vi "ICR_Setup_Sequence.vi"(8 "error in (no error)":errorcluster, 9 "QMH UI Cluster":variant, 11 "QMH ICR Cluster":T1) -> (0 "error out":errorcluster, 3 "QMH ICR Cluster":T1)   [LabVIEW 2024]
doc: "This VI updates the indicators of the ICR panel according to the parameters setup by the user and the controls in the UI main panel.\n\n1. The indicators are passed by reference through the QMH ICR Cluster.\n2. Their values are updated with the QMH UI Cluster parameters.\n3. The QMH ICR Cluster given in output contains the updated indicators."
uses:
  controls/QMH_ICR_Cluster.ctl
  controls/HARDWARE_Resources.ctl
  controls/PROCESSING_Inputs.ctl
  controls/LOOPS_Inputs.ctl
  controls/OPO_Inputs.ctl
  controls/QMH_UI_Cluster.ctl
  controls/QMH_UI_References.ctl
  controls/QMH_UI_Report.ctl
  controls/QMH_UI_Command.ctl
  controls/QMH_ICR_Command.ctl
  controls/QMH_Status.ctl
  controls/EXPERT_Inputs.ctl
  controls/DIGIT_5122_Inputs.ctl
  <instrlib>/niScope/Controls/niScope trigger source.ctl
  controls/HSDIO_6541_Inputs.ctl
  <instrlib>/niHSDIO/niHSDIO.llb/niHSDIO_ctl Trigger Source Values (Ring).ctl
  controls/SOFTWARE_Inputs.ctl
  controls/AO_6711_Inputs.ctl
  controls/AWG_5421_Inputs.ctl
  <instrlib>/niFgen/niFgen.llb/niFgen_ctl Trigger Source Values (Ring).ctl
  controls/XML_Inputs.ctl
  controls/SEQUENCE_Inputs.ctl
  controls/EXCIT_Inputs.ctl
  controls/DATA_Inputs.ctl
  controls/TIMING_Inputs.ctl
  controls/TRAPPING_Inputs.ctl
  controls/EXPERT_Path_Selector.ctl
  controls/EXPERIMENT_Inputs.ctl
  controls/LASER_Inputs.ctl
  controls/LAMP_Inputs.ctl
  controls/GAS_Inputs.ctl
  Global_Variables.vi
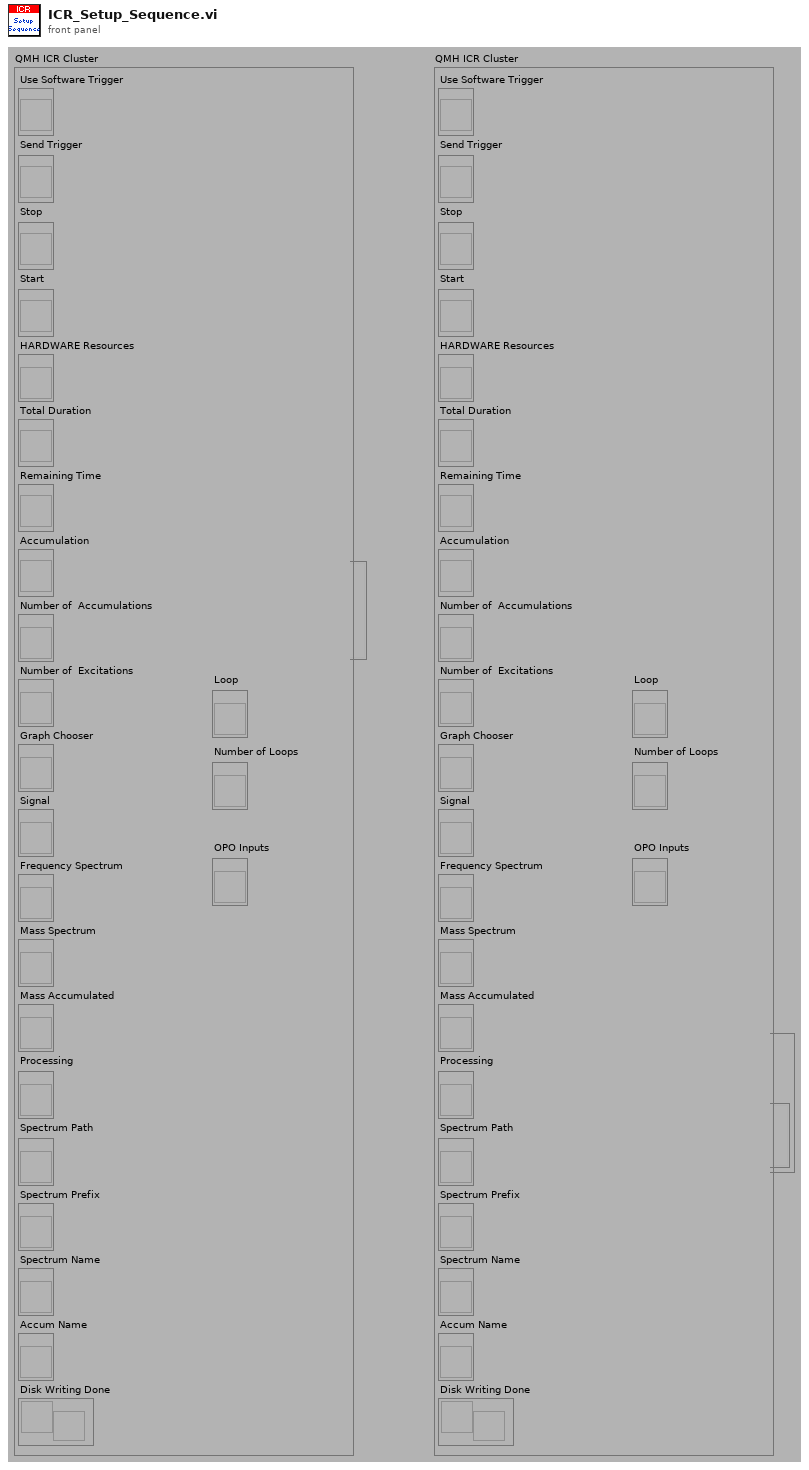
[diagram p1: front panel]
types:
  T1 = typedef "QMH_ICR_Cluster.ctl" = cluster{"Use Software Trigger":refnum<vi>, "Send Trigger":refnum<vi>, "Stop":refnum<vi>, "Start":refnum<vi>, "HARDWARE Resources":refnum<vi>, "Total Duration":refnum<vi>, "Remaining Time":refnum<vi>, "Accumulation":refnum<vi>, "Number of  Accumulations":refnum<vi>, "Number of  Excitations":refnum<vi>, "Graph Chooser":refnum<vi>, "Signal":refnum<vi>, "Frequency Spectrum":refnum<vi>, "Mass Spectrum":refnum<vi>, "Mass Accumulated":refnum<vi>, "Processing":refnum<vi>, "Spectrum Path":refnum<vi>, "Spectrum Prefix":refnum<vi>, "Spectrum Name":refnum<vi>, "Accum Name":refnum<vi>, "Disk Writing Done":refnum<notifier>, "Loop":refnum<vi>, "Number of Loops":refnum<vi>, "OPO Inputs":refnum<vi>}
  T2 = typedef "EXPERT_Path_Selector.ctl" = enum16{"Application", "Resources", "Data", "XML", "XML Saved", "Load Directory"}
  T3 = typedef "EXPERIMENT_Inputs.ctl" = cluster{"Setup":string, "Date":string, "User Name":string, "Comment":string, "Experiment Procedures":string[], "Chemical Source":string, "Sample Components":string[], "Species":string[], "Laser 1":T4, "Laser 2":T4, "Laser 3":T4, "Laser 4":T4, "Laser 5":T4, "Lamp 1":T5, "Lamp 2":T5, "Gas 1":T6, "Gas 2":T6, "Gas 3":T6, "Gas 4":T6, "Gas 5":T6}
  T4 = typedef "LASER_Inputs.ctl" = cluster{"Used":bool, "Name":string, "Wavelength":dbl, "Energy":dbl}
  T5 = typedef "LAMP_Inputs.ctl" = cluster{"Used":bool, "Name":string, "Wavelength":dbl, "Attenuation":dbl}
  T6 = typedef "GAS_Inputs.ctl" = cluster{"Used":bool, "Name":string, "Pressure":dbl}
  T7 = typedef "SEQUENCE_Inputs.ctl" = cluster{"EXCIT Inputs":T8, "DATA Inputs":T9, "TIMING Inputs":T10, "PROCESSING Inputs":T11, "TRAPPING Inputs":T12}
  T8 = typedef "EXCIT_Inputs.ctl" = cluster{"Number of Excitations":i32, "Script Text":string, "Table of Waveforms":string[]}
  T9 = typedef "DATA_Inputs.ctl" = cluster{"Record Length":i32, "Sample Rate":dbl, "Data Type":u8, "Vertical Range":dbl, "Acquisition Duration":dbl}
  T10 = typedef "TIMING_Inputs.ctl" = cluster{"Number of Acquisitions ":i16, "Number of Accumulations":i16, "Table of Waveforms":string[], "Script Text":string}
  T11 = typedef "PROCESSING_Inputs.ctl" = cluster{"Reference Mass":dbl, "Cyclotron Freq":dbl, "Magnetron Freq":dbl}
  T12 = typedef "TRAPPING_Inputs.ctl" = cluster{"Number of Channels":i32, "Init Values":dbl[], "Opening Values":dbl[], "Trapping Values":dbl[], "Emptying Values":dbl[], "Adiabatic ON":bool, "Adiabatic Duration":i32, "Adiabatic Waveforms":string[], "Ions Refill ON":bool, "Number of Ions Refills":i32}
  T13 = typedef "EXPERT_Inputs.ctl" = cluster{"DIGIT 5122 Inputs":T14, "HSDIO 6541 Inputs":T16, "SOFTWARE Inputs":T18, "AO 6711 Inputs":T19, "AWG 5421 Inputs":T20, "XML Inputs":T22}
  T14 = typedef "DIGIT_5122_Inputs.ctl" = cluster{"Sample Rate":dbl, "Resource Name":refnum<k15>, "Channel Name":string, "Trigger Source":T15, "Vertical Range":dbl, "Trigger Level":dbl}
  T15 = typedef "niScope trigger source.ctl" = string
  T16 = typedef "HSDIO_6541_Inputs.ctl" = cluster{"Resource Name":refnum<k15>, "Clock Rate":dbl, "Trigger Source":T17}
  T17 = typedef "niHSDIO_ctl Trigger Source Values (Ring).ctl" = string
  T18 = typedef "SOFTWARE_Inputs.ctl" = cluster{"Application Directory":path, "Software Version":string, "Data Path":path, "XML Path":path, "XML File Filter":string, "XML Saved Path":path, "Excit Scripts Path":path, "Excit Scripts File Filter":string, "Excit Waveforms Path":path, "Excit Waveforms File Filter":string, "Timing Scripts Path":path, "Timing Scripts File Filter":string, "Timing Waveforms Path":path, "Timing Waveforms File Filter":string, "Trapping Waveforms Path":path, "Trapping Waveforms File Filter":string}
  T19 = typedef "AO_6711_Inputs.ctl" = cluster{"Physical Channels":tag, "Min Voltage":dbl, "Max Voltage":dbl, "Trigger Source":tag, "Counter":tag}
  T20 = typedef "AWG_5421_Inputs.ctl" = cluster{"Resource Name":refnum<k15>, "Sample Rate":dbl, "Trigger Type":u16, "Trigger Source":T21, "Waveform Gain":dbl, "Digital Filter ON":bool}
  T21 = typedef "niFgen_ctl Trigger Source Values (Ring).ctl" = string
  T22 = typedef "XML_Inputs.ctl" = cluster{"Version Tag Name":string, "Version String":string}
  T23 = typedef "QMH_UI_Cluster.ctl" = cluster{"QMH UI References":T24, "QMH UI Report":T25}
  T24 = typedef "QMH_UI_References.ctl" = cluster{"Refnum Load":refnum<vi>, "Refnum Save As":refnum<vi>, "Refnum Start":refnum<vi>, "Refnum Exit":refnum<vi>, "Refnum Tabs":refnum<vi>, "Refnum SPECTRUM":refnum<vi>, "Refnum EXPERIMENT":refnum<vi>, "Refnum VOLTAGES":refnum<vi>, "Refnum SEQUENCE":refnum<vi>, "Refnum EXPERT":refnum<vi>, "Refnum LOOPS":refnum<vi>, "Refnum EXCIT Table":refnum<vi>, "Refnum TIMING Table":refnum<vi>, "Refnum CHANGE Experiment":refnum<vi>, "Refnum CHANGE Voltages":refnum<vi>, "Refnum CHANGE Sequence":refnum<vi>, "Refnum CHANGE Expert":refnum<vi>, "Refnum CHANGE Loops":refnum<vi>, "Refnum CHANGE Scientist":refnum<vi>, "Refnum PIL Status":refnum<vi>}
  T25 = typedef "QMH_UI_Report.ctl" = cluster{"UI Status":T26, "ICR Status":T27, "QMH Status":T28}
  T26 = typedef "QMH_UI_Command.ctl" = enum16{"Initialize", "UI Load", "UI Save", "UI Save As", "UI Change Experiment", "UI Change Voltages", "UI Change Sequence", "UI Change Expert", "UI Change Loops", "UI Change Scientist", "Ready to Start", "UI Start", "Waiting for ICR", "UI Exit", "Update Experiment", "Update Report", "Update ICR Status", "Waiting for User"}
  T27 = typedef "QMH_ICR_Command.ctl" = enum16{"Initialize", "Sequence Loop Setup", "Sequence Setup", "ICR Start", "ICR Stop", "Hardware Setup", "Next Sequence Loop", "Next Accumulation", "Waiting for Trigger", "Sequence Started", "Sequence Finished", "Sequence Loop Done", "Writing Data", "Hardware Reset", "Exit"}
  T28 = typedef "QMH_Status.ctl" = enum16{"Init", "Loading", "Setup", "Ready to Start", "Started", "Idle"}
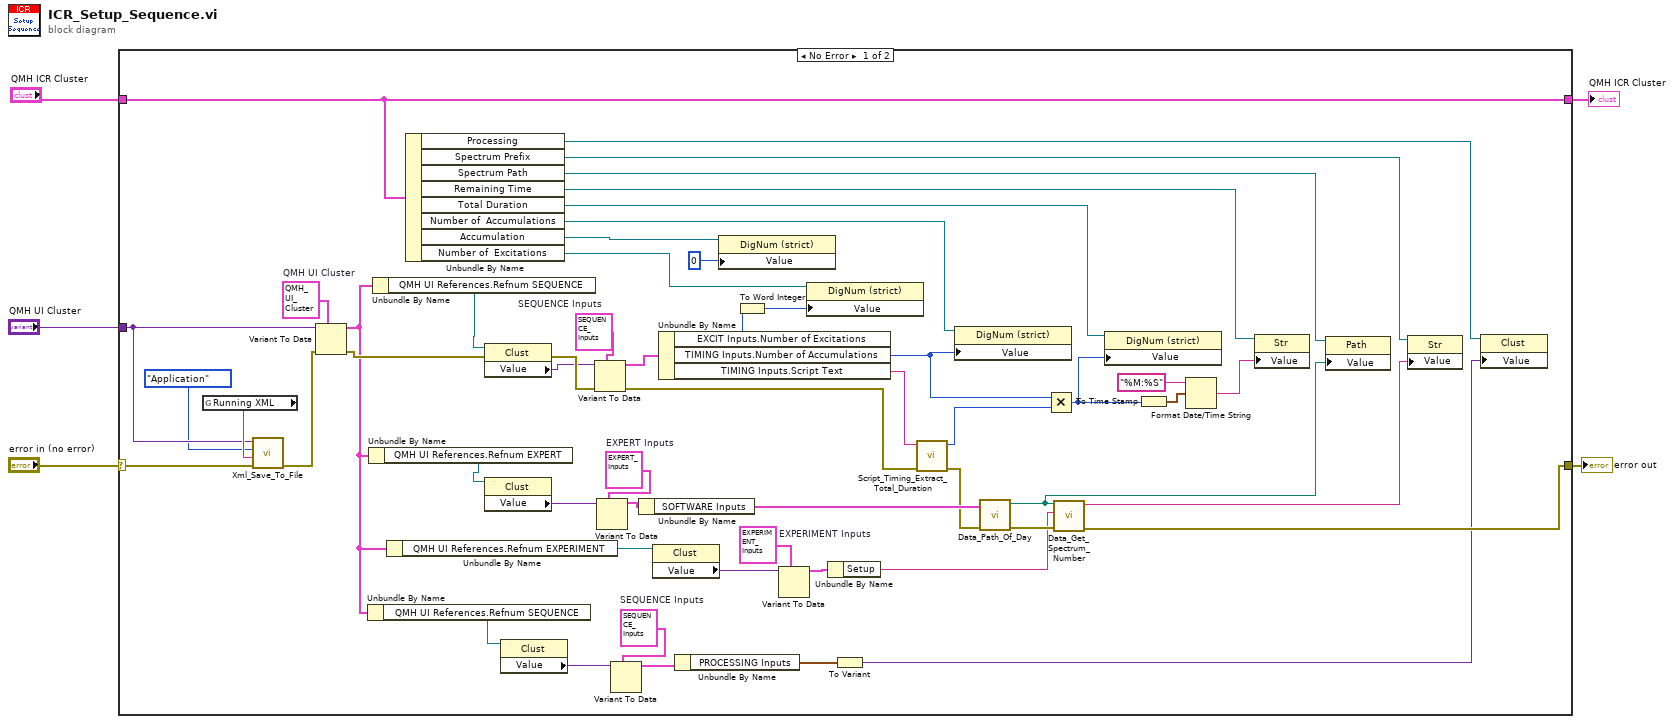
[diagram p0: block diagram]
diagram:
  n1 = case shown="No Error" "error in (no error)" {
    selector: "error in (no error)" -> [w44 w61]
    tunnel: [w29 w61] -> w5
    tunnel: "QMH UI Cluster" -> [w18 _]
    tunnel: "QMH ICR Cluster" -> [w53 w60]
    tunnel: [w53 w60] -> w1
    frame No Error {
      w14 = T3 {"Setup"="", "Date"="", "User Name"="", "Comment"="", "Experiment Procedures"=[], "Chemical Source"="", "Sample Components"=[], "Species"=[], "Laser 1"={"Used"=TRUE, "Name"="Spectroscopy", "Wavelength"=1000.0, "Energy"=25.0}, "Laser 2"={"Used"=TRUE, "Name"="Spectroscopy", "Wavelength"=1000.0, "Energy"=25.0}, "Laser 3"={"Used"=TRUE, "Name"="Spectroscopy", "Wavelength"=1000.0, "Energy"=25.0}, "Laser 4"={"Used"=TRUE, "Name"="Spectroscopy", "Wavelength"=1000.0, "Energy"=25.0}, "Laser 5"={"Used"=TRUE, "Name"="Spectroscopy", "Wavelength"=1000.0, "Energy"=25.0}, "Lamp 1"={"Used"=TRUE, "Name"="Spectroscopy", "Wavelength"=1000.0, "Attenuation"=25.0}, "Lamp 2"={"Used"=TRUE, "Name"="Spectroscopy", "Wavelength"=1000.0, "Attenuation"=25.0}, "Gas 1"={"Used"=TRUE, "Name"="Spectroscopy", "Pressure"=1000.0}, "Gas 2"={"Used"=TRUE, "Name"="Spectroscopy", "Pressure"=1000.0}, "Gas 3"={"Used"=TRUE, "Name"="Spectroscopy", "Pressure"=1000.0}, "Gas 4"={"Used"=TRUE, "Name"="Spectroscopy", "Pressure"=1000.0}, "Gas 5"={"Used"=TRUE, "Name"="Spectroscopy", "Pressure"=1000.0}}  # EXPERIMENT Inputs
      w24 = T7 {"EXCIT Inputs"={"Number of Excitations"=0, "Script Text"="", "Table of Waveforms"=[]}, "DATA Inputs"={"Record Length"=0, "Sample Rate"=0.0, "Data Type"=0, "Vertical Range"=0.0, "Acquisition Duration"=0.0}, "TIMING Inputs"={"Number of Acquisitions "=0, "Number of Accumulations"=0, "Table of Waveforms"=[], "Script Text"=""}, "PROCESSING Inputs"={"Reference Mass"=0.0, "Cyclotron Freq"=0.0, "Magnetron Freq"=0.0}, "TRAPPING Inputs"={"Number of Channels"=0, "Init Values"=[], "Opening Values"=[], "Trapping Values"=[], "Emptying Values"=[], "Adiabatic ON"=FALSE, "Adiabatic Duration"=0, "Adiabatic Waveforms"=[], "Ions Refill ON"=FALSE, "Number of Ions Refills"=0}}  # SEQUENCE Inputs
      w36 = T13 {"DIGIT 5122 Inputs"={"Sample Rate"=10000.0, "Resource Name"="DIGIT_5122", "Channel Name"="0", "Trigger Source"="VAL_EXTERNAL", "Vertical Range"=10.0, "Trigger Level"=3.0}, "HSDIO 6541 Inputs"={"Resource Name"="HSDIO_6541", "Clock Rate"=1000000.0, "Trigger Source"="PFI0"}, "SOFTWARE Inputs"={"Application Directory"=path "D:/S.O.F.T.S/LABVIEW/PIL", "Software Version"="1.0.0", "Data Path"=path "D:/PIRENEA/DATA", "XML Path"=path "D:/PIRENEA/DATA", "XML File Filter"="*.xml", "XML Saved Path"=path "D:/PIRENEA/DATA", "Excit Scripts Path"=path "D:/PIRENEA/EXCIT_SCRIPTS", "Excit Scripts File Filter"="*.txt", "Excit Waveforms Path"=path "D:/PIRENEA/EXCIT_WFMS", "Excit Waveforms File Filter"="*.bin", "Timing Scripts Path"=path "D:/PIRENEA/SEQUENCE_SCRIPTS", "Timing Scripts File Filter"="*.txt", "Timing Waveforms Path"=path "D:/PIRENEA/SEQUENCE_WFMS", "Timing Waveforms File Filter"="*.bin", "Trapping Waveforms Path"=path "D:/PIRENEA/TRAPPING_WFMS", "Trapping Waveforms File Filter"="*.bin"}, "AO 6711 Inputs"={"Physical Channels"="AO_6711/ao0:3", "Min Voltage"=-10.0, "Max Voltage"=10.0, "Trigger Source"="/AO_6711/PFI0", "Counter"="AO_6711/ctr0"}, "AWG 5421 Inputs"={"Resource Name"="AWG_5421", "Sample Rate"=20000000.0, "Trigger Type"=2, "Trigger Source"="PFI0", "Waveform Gain"=0.31, "Digital Filter ON"=TRUE}, "XML Inputs"={"Version Tag Name"="XML_Version", "Version String"="1.0"}}  # EXPERT Inputs
      w57 = T7 {"EXCIT Inputs"={"Number of Excitations"=0, "Script Text"="", "Table of Waveforms"=[]}, "DATA Inputs"={"Record Length"=0, "Sample Rate"=0.0, "Data Type"=0, "Vertical Range"=0.0, "Acquisition Duration"=0.0}, "TIMING Inputs"={"Number of Acquisitions "=0, "Number of Accumulations"=0, "Table of Waveforms"=[], "Script Text"=""}, "PROCESSING Inputs"={"Reference Mass"=0.0, "Cyclotron Freq"=0.0, "Magnetron Freq"=0.0}, "TRAPPING Inputs"={"Number of Channels"=0, "Init Values"=[], "Opening Values"=[], "Trapping Values"=[], "Emptying Values"=[], "Adiabatic ON"=FALSE, "Adiabatic Duration"=0, "Adiabatic Waveforms"=[], "Ions Refill ON"=FALSE, "Number of Ions Refills"=0}}  # SEQUENCE Inputs
      w59 = T23 {"QMH UI References"={"Refnum Load"=refnum, "Refnum Save As"=refnum, "Refnum Start"=refnum, "Refnum Exit"=refnum, "Refnum Tabs"=refnum, "Refnum SPECTRUM"=refnum, "Refnum EXPERIMENT"=refnum, "Refnum VOLTAGES"=refnum, "Refnum SEQUENCE"=refnum, "Refnum EXPERT"=refnum, "Refnum LOOPS"=refnum, "Refnum EXCIT Table"=refnum, "Refnum TIMING Table"=refnum, "Refnum CHANGE Experiment"=refnum, "Refnum CHANGE Voltages"=refnum, "Refnum CHANGE Sequence"=refnum, "Refnum CHANGE Expert"=refnum, "Refnum CHANGE Loops"=refnum, "Refnum CHANGE Scientist"=refnum, "Refnum PIL Status"=refnum}, "QMH UI Report"={"UI Status"=enum."Initialize", "ICR Status"=enum."Initialize", "QMH Status"=enum."Init"}}  # QMH UI Cluster
      n2 = global read "Global_Variables.vi" "Running XML"() -> (w19:string)
      n3 = call "Xml_Save_To_File.vi"("error in (no error)"=w44, "Filename"=w19, "EXPERT Path Selector"=EXPERT_Path_Selector."Application", "Variant"=w18) -> ("error out"=w43:errorcluster)  [unwired: 7 in]
      n4 = Variant To Data(error in=w43, type=w59, Variant=w18) -> (data=w6:T23, error out=w46:errorcluster)
      n5 = Unbundle By Name(w6) -> ("QMH UI References.Refnum SEQUENCE"=w25:refnum<vi>)
      n6 = Unbundle By Name(w6) -> ("QMH UI References.Refnum EXPERT"=w38:refnum<vi>)
      n7 = Unbundle By Name(w6) -> ("QMH UI References.Refnum SEQUENCE"=w55:refnum<vi>)
      n8 = Unbundle By Name(w6) -> ("QMH UI References.Refnum EXPERIMENT"=w16:refnum<vi>)
      n9 = Unbundle By Name(w53) -> ("Processing"=w22:refnum<vi>, "Spectrum Prefix"=w28:refnum<vi>, "Spectrum Path"=w32:refnum<vi>, "Remaining Time"=w48:refnum<vi>, "Total Duration"=w52:refnum<vi>, "Number of  Accumulations"=w47:refnum<vi>, "Accumulation"=w42:refnum<vi>, "Number of  Excitations"=w10:refnum<vi>)
      n10 = property class="Clust"(reference=w55, error in=w46) -> (error out=w58:errorcluster, "Value"=w56:variant)  [unwired: 1 out]
      n11 = property class="Clust"(reference=w38) -> ("Value"=w37:variant)  [unwired: 1 in, 2 out]
      n12 = property class="Clust"(reference=w25) -> ("Value"=w26:variant)  [unwired: 1 in, 2 out]
      n13 = Variant To Data(error in=w58, type=w57, Variant=w56) -> (data=w54:T7, error out=w45:errorcluster)
      n14 = Variant To Data(type=w36, Variant=w37) -> (data=w35:T13)  [unwired: 1 in, 1 out]
      n15 = Variant To Data(type=w24, Variant=w26) -> (data=w23:T7)  [unwired: 1 in, 1 out]
      n16 = Unbundle By Name(w35) -> ("SOFTWARE Inputs"=w34:T18)
      n17 = property class="Clust"(reference=w16) -> ("Value"=w15:variant)  [unwired: 1 in, 2 out]
      n18 = Unbundle By Name(w54) -> ("EXCIT Inputs.Number of Excitations"=w9:i32, "TIMING Inputs.Number of Accumulations"=w39:i16, "TIMING Inputs.Script Text"=w7:string)
      n19 = Unbundle By Name(w23) -> ("PROCESSING Inputs"=w21:T11)
      n20 = property class="DigNum (strict)"(reference=w42, "Value"=i16 0 ("Valeur")) -> ()  [unwired: 1 in, 2 out]
      n21 = To Word Integer(number=w9) -> (16bit integer=w8:i16)
      n22 = Variant To Data(type=w14, Variant=w15) -> (data=w13:T3)  [unwired: 1 in, 1 out]
      n23 = property class="DigNum (strict)"(reference=w10, "Value"=w8) -> ()  [unwired: 1 in, 2 out]
      n24 = Unbundle By Name(w13) -> ("Setup"=w12:string)
      n25 = To Variant(anything=w21) -> (Variant=w20:variant)
      n26 = call "Script_Timing_Extract_Total_Duration.vi"("error in (no error)"=w45, "Script"=w7) -> ("error out"=w30:errorcluster, "Total duration (s)"=w11:i32)  [unwired: 8 in]
      n27 = property class="DigNum (strict)"(reference=w47, "Value"=w39) -> ()  [unwired: 1 in, 2 out]
      n28 = call "Data_Path_Of_Day.vi"("error in (no error)"=w30, "SOFTWARE Inputs"=w34) -> ("error out"=w33:errorcluster, "Path of the Day"=w31:path)  [unwired: 8 in]
      n29 = Multiply(x=w39, y=w11) -> (x*y=w40:i32)
      n30 = call "Data_Get_Spectrum_Number.vi"("error in (no error)"=w33, "Setup"=w12, "Path of the Day"=w31) -> ("error out"=w29:errorcluster, "Next Spectrum Number"=w27:string)  [unwired: 6 in, 1 out]
      n31 = property class="DigNum (strict)"(reference=w52, "Value"=w40) -> ()  [unwired: 1 in, 2 out]
      n32 = To Time Stamp(1:w40) -> (0:w51:timestamp)
      n33 = Format Date/Time String(time format string (%c)="%M:%S" ("chaîne de format de l'heure (%c)"), seconds (now)=w51) -> (date/time string=w50:string)  [unwired: 1 in]
      n34 = property class="Str"(reference=w48, "Value"=w50) -> ()  [unwired: 1 in, 2 out]
      n35 = property class="Path"(reference=w32, "Value"=w31) -> ()  [unwired: 1 in, 2 out]
      n36 = property class="Str"(reference=w28, "Value"=w27) -> ()  [unwired: 1 in, 2 out]
      n37 = property class="Clust"(reference=w22, "Value"=w20) -> ()  [unwired: 1 in, 2 out]
    }
    frame Error {
    }
  }
  "error out" <- w5
  "QMH ICR Cluster" <- w1
